vi "Add Routing Channel.vi"(8 "error in (no error)":errorcluster, 9 "States and Connections":T1, 10 "Channel Name":string, 11 "Routes Ref in":T4 format="%.0x") -> (0 "error out":errorcluster, 2 "Channel Ref":T4 format="%.0x", 3 "Routes Ref out":T4 format="%.0x")   [LabVIEW 2017, in "Switch Scripting.lvlib"]
uses:
  Switch Scripting.lvlib
  <vilib>/NI Veristand/Custom Device API/Custom Device Item Ref.ctl
  Channel States.ctl
  Routing State.ctl
  Connection.ctl
  <vilib>/NI Veristand/Custom Device API/Custom Device Channel.ctl
  <vilib>/NI Veristand/Custom Device API/Custom Device Channel Type.ctl
  <vilib>/NI VeriStand/Custom Device API/Custom Device API.lvlib
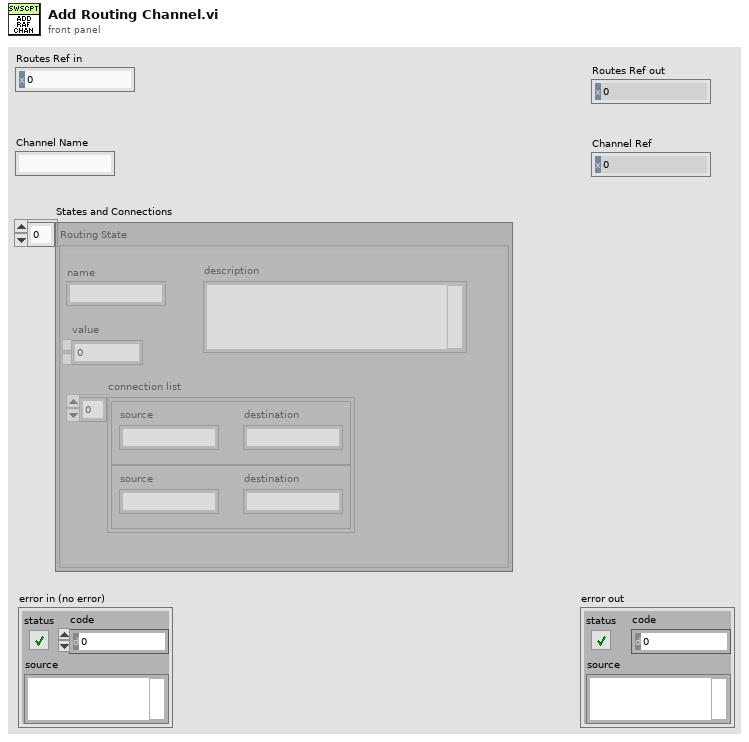
[diagram p1: front panel]
types:
  T1 = typedef "Switch Scripting.lvlib/Channel States.ctl" = T2[]
  T2 = typedef "Switch Scripting.lvlib/Routing State.ctl" = cluster{"name":string, "description":string, "value":i32, "connection list":T3[]}
  T3 = typedef "Switch Scripting.lvlib/Connection.ctl" = cluster{"source":string, "destination":string}
  T4 = typedef "Custom Device API.lvlib/Custom Device Item Ref.ctl" = u64
  T5 = typedef "Custom Device API.lvlib/Custom Device Channel.ctl" = cluster{"Type":T6, "Units":string, "Default Value":dbl, "Faultable":bool, "Scalable":bool}
  T6 = typedef "Custom Device API.lvlib/Custom Device Channel Type.ctl" = enum16{"Input", "Output"}
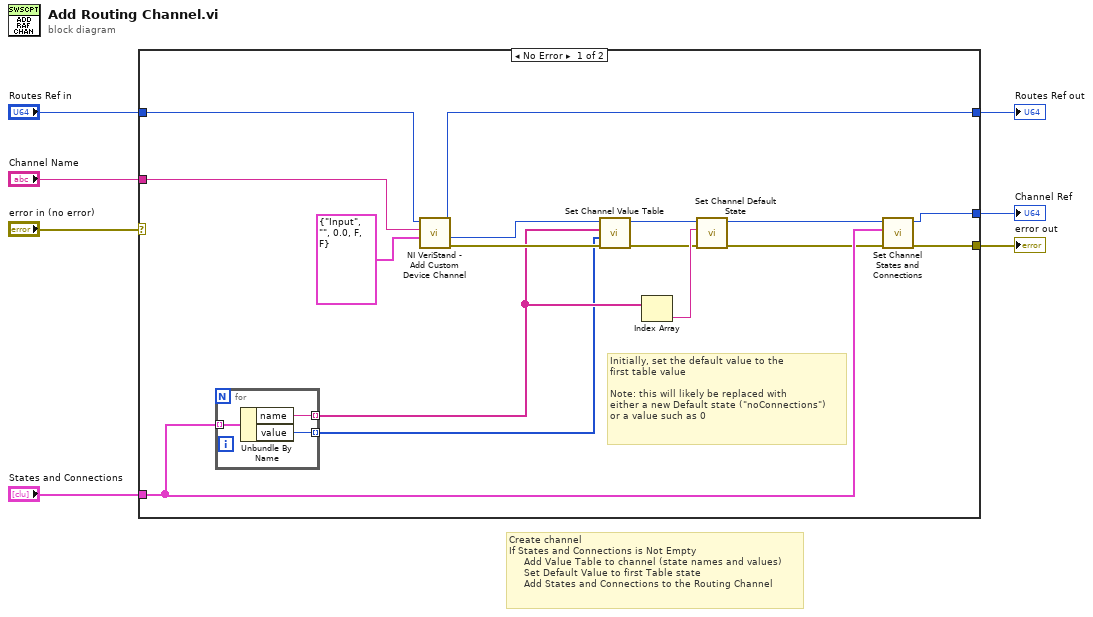
[diagram p0: block diagram]
diagram:
  # "Create channel\nIf States and Connections is Not Empty\n     Add Value Table to channel (state names and values)\n     Set Default Value to first Table state\n     Add States and Connections to the Routing Channel"
  n1 = case shown="No Error" "error in (no error)" {
    selector: "error in (no error)" -> [_ w27]
    tunnel: [w21 w27] -> w7
    tunnel: [w16 w26] -> w6
    tunnel: "Routes Ref in" -> [w17 w26]
    tunnel: "Channel Name" -> [w22 _]
    tunnel: [w18 _] -> w2
    tunnel: "States and Connections" -> [w20 _]
    frame No Error {
      # "Initially, set the default value to the \nfirst table value\n\nNote: this will likely be replaced with\neither a new Default state (\"noConnections\")\nor a value such as 0"
      n2 = for {
        tunnel: w20 -> [w25] mode=indexing
        tunnel: [w24] -> w9 mode=indexing
        tunnel: [w23] -> w8 mode=indexing
        n3 = Unbundle By Name(w25) -> ("name"=w24:string, "value"=w23:i32)
      }
      n4 = call <vilib>:"NI VeriStand - Add Custom Device Channel.vi"("Channel"=T5 {"Type"=enum."Input", "Units"="", "Default Value"=0.0, "Faultable"=FALSE, "Scalable"=FALSE}, "Channel Name"=w22, "Parent Ref in"=w17) -> ("error out"=w19:errorcluster, "Channel Ref"=w15:T4, "Parent Ref out"=w16:T4)  [unwired: 5 in, 1 out]
      n5 = call "Set Channel Value Table.vi"("error in (no error)"=w19, "Values"=w8, "States"=w9, "Channel Ref in"=w15) -> ("error out"=w12:errorcluster)  [unwired: 6 in, 1 out]
      n6 = Index Array(array=w9) -> (element=w13:string)  [unwired: 1 in]
      n7 = call "Set Channel Default State.vi"("error in (no error)"=w12, "State"=w13, "Channel Ref in"=w15) -> ("error out"=w11:errorcluster, "Channel Ref out"=w14:T4)  [unwired: 7 in]
      n8 = call "Set Channel States and Connections.vi"("error in (no error)"=w11, "Routing Channel States"=w20, "Channel Ref in"=w14) -> ("error out"=w21:errorcluster, "Channel Ref out"=w18:T4)  [unwired: 7 in]
    }
    frame Error {
    }
  }
  "error out" <- w7
  "Routes Ref out" <- w6
  "Channel Ref" <- w2
